vi "Display Biometry Ascan.vi"(8 "错误常量":errorcluster, 9 "L_Or_R":string, 10 "Measure_No":i32, 11 "connection reference":T1) -> (0 "error out":errorcluster)   [LabVIEW 2015, in "Browse.lvlib"]
uses:
  Browse.lvlib
  <vilib>/addons/database/Connection.llb/Conn ObjectReference.ctl
  Support/Display Biometry Ascan State.ctl
  Support/Biometry Ascan UI Data.ctl
  Sub VIs/Database Processing/Database Processing.lvlib
  Sub VIs/Utility VIs/Utility VIs.lvlib
  <vilib>/addons/database/NI_Database_API.lvlib
panel:
  out "Ascan":dbl[][](graph)
  out "Parameter":string[][](table)
  in  "停止按钮":bool
  out "状态栏":string
  # "眼轴参数"
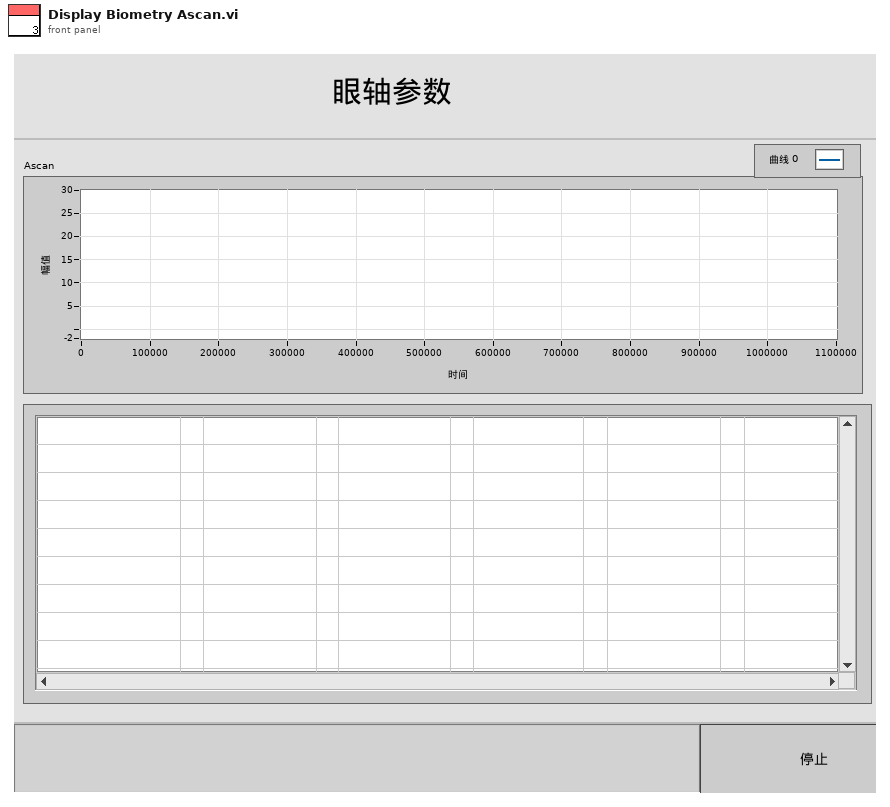
[diagram p1: front panel]
types:
  T1 = typedef "NI_Database_API.lvlib/Conn ObjectReference.ctl" = refnum<k1>
  T2 = typedef "Browse.lvlib/Biometry Ascan UI Data.ctl" = cluster{"Parameter引用句柄":refnum<vi>, "状态栏引用句柄":refnum<vi>, "退出引用句柄":refnum<vi>, "Asacn引用句柄":refnum<vi>}
  T3 = typedef "Browse.lvlib/Display Biometry Ascan State.ctl" = enum16{"Initialize", "Connect Database", "Update Biometry Ascan Single", "Update Biometry Ascan multiple", "Update Biometry Parameter", "Wait For Event", "Exit"}
  T4 = typedef "LVPoint32TypeDef.ctl" = cluster{"Horizontal":i32, "Vertical":i32}
  T5 = typedef "LVRowAndColumnTypeDef.ctl" = cluster{"Row":i32, "Column":i32}
  T6 = typedef "Database Processing.lvlib/Biometry Data Path.ctl" = cluster{"Measure_ID":i64, "Ascan_data_Original":string, "picture_pupil_Original":string, "picture_WTW_Original":string, "Ascan_data_Processing":string, "picture_pupil_Processing":string, "picture_WTW_Processing":string, "picture_Processing_K":string, "picture_Processing_ALL":string}
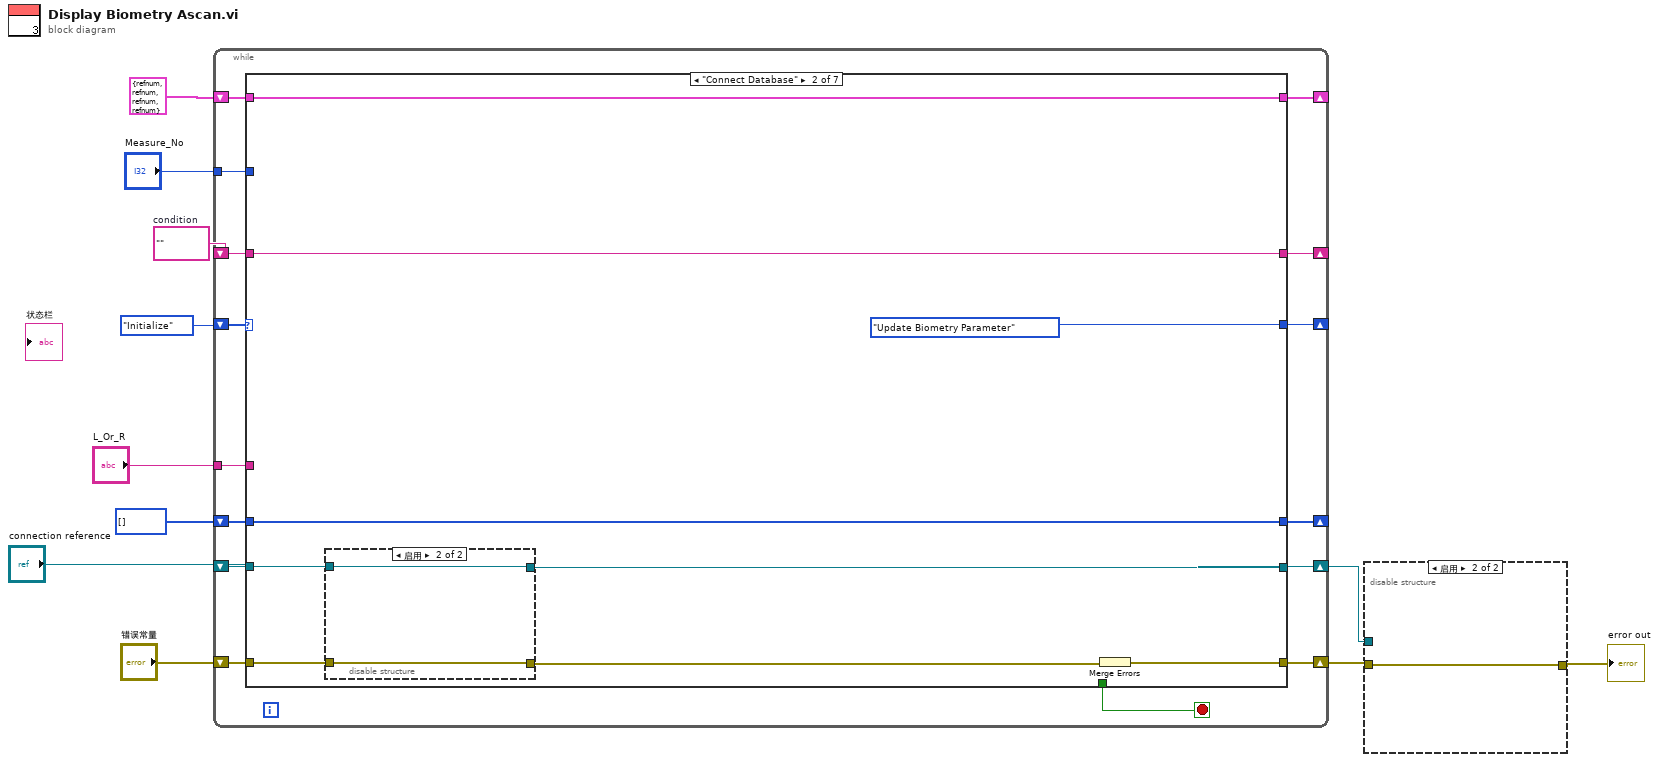
[diagram p0: block diagram]
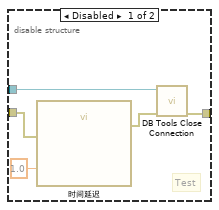
[diagram p2: hidden frame]
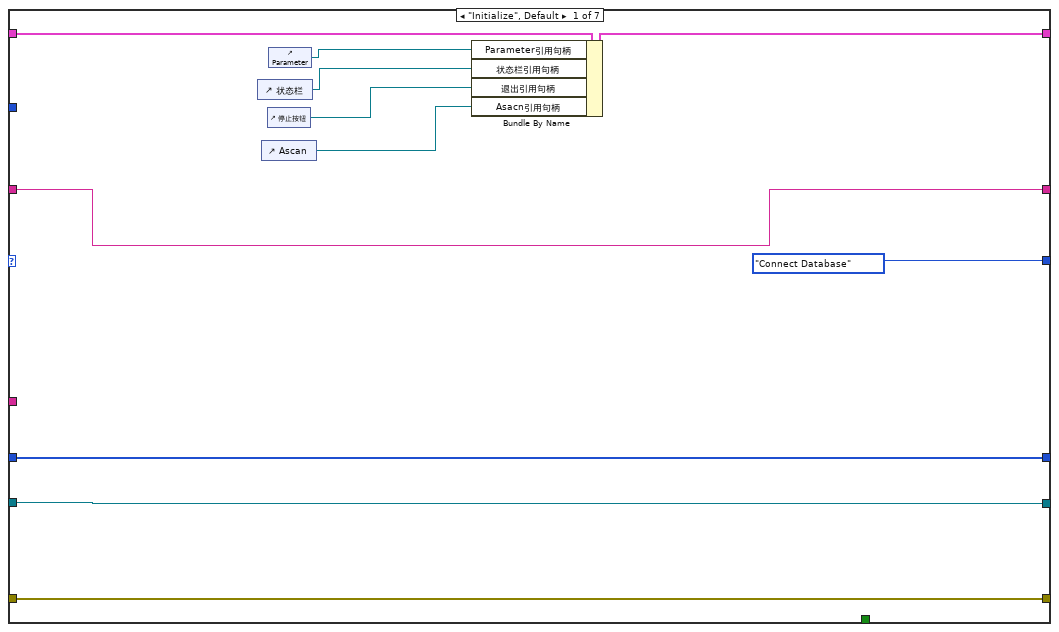
[diagram p3: hidden frame]
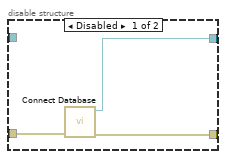
[diagram p4: hidden frame]
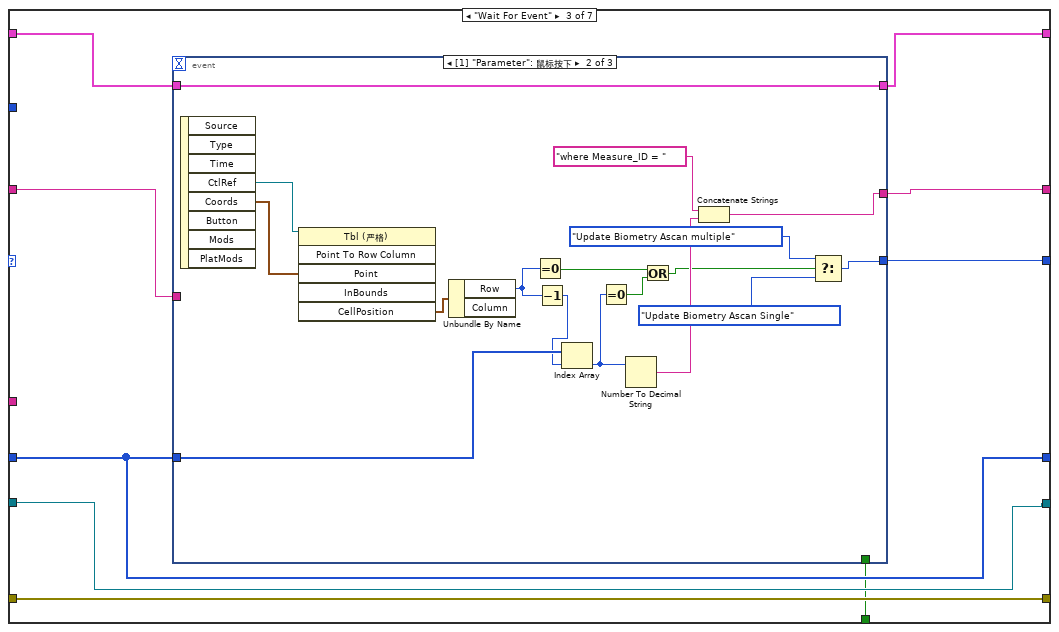
[diagram p5: hidden frame]
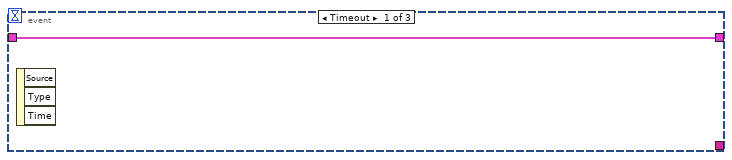
[diagram p6: hidden frame]
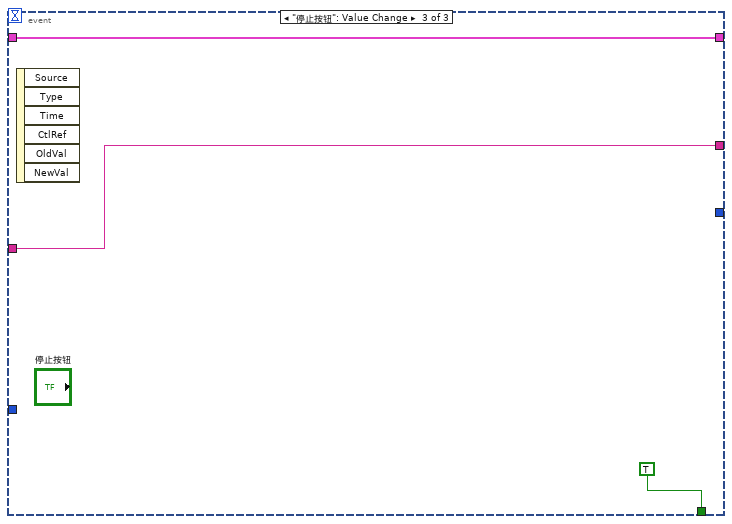
[diagram p7: hidden frame]
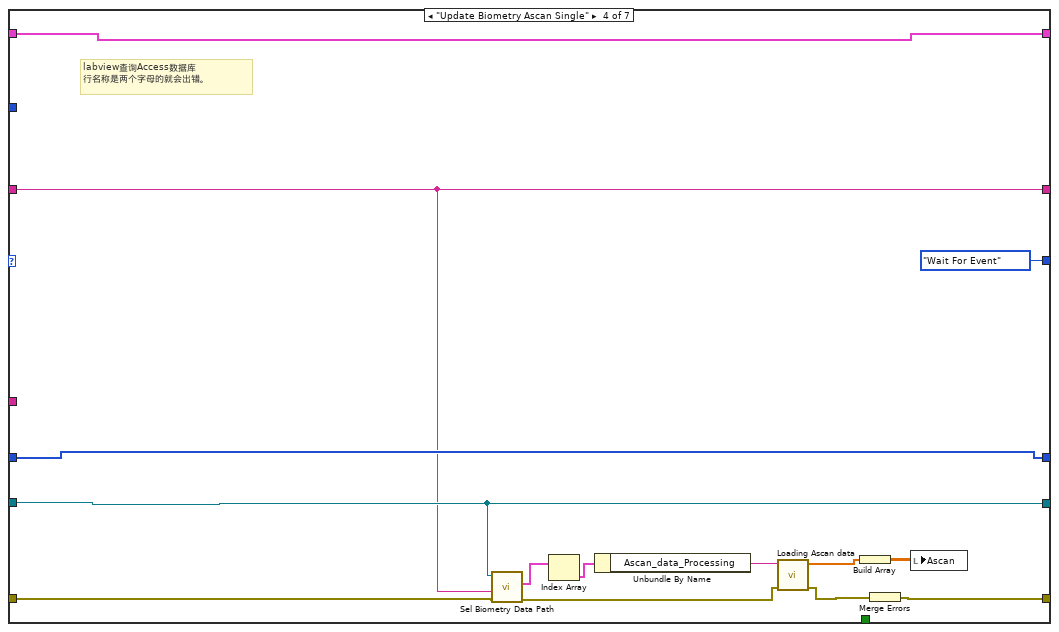
[diagram p8: hidden frame]
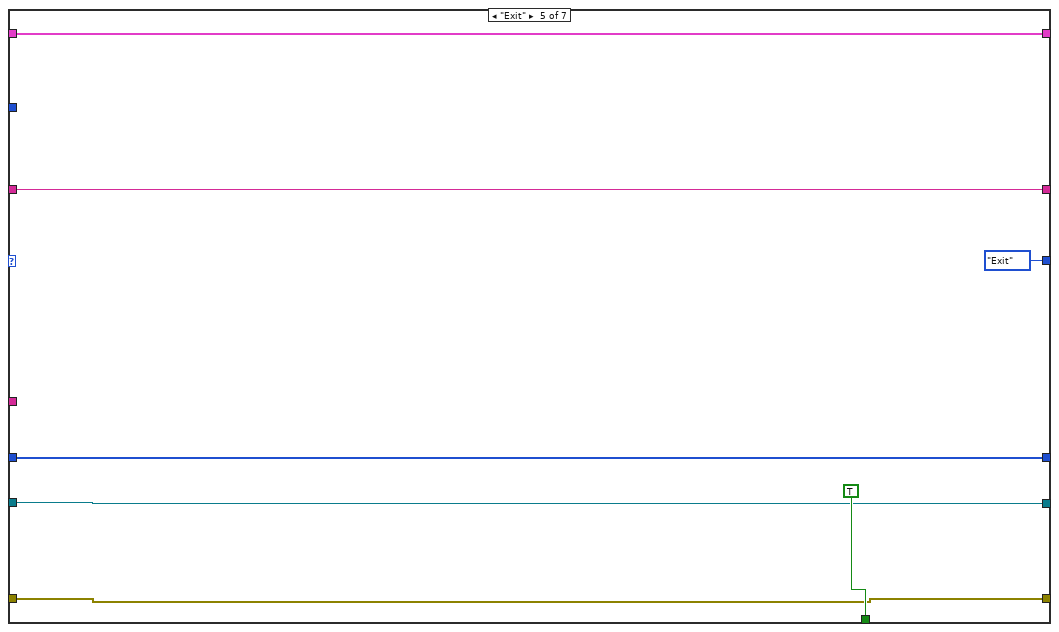
[diagram p9: hidden frame]
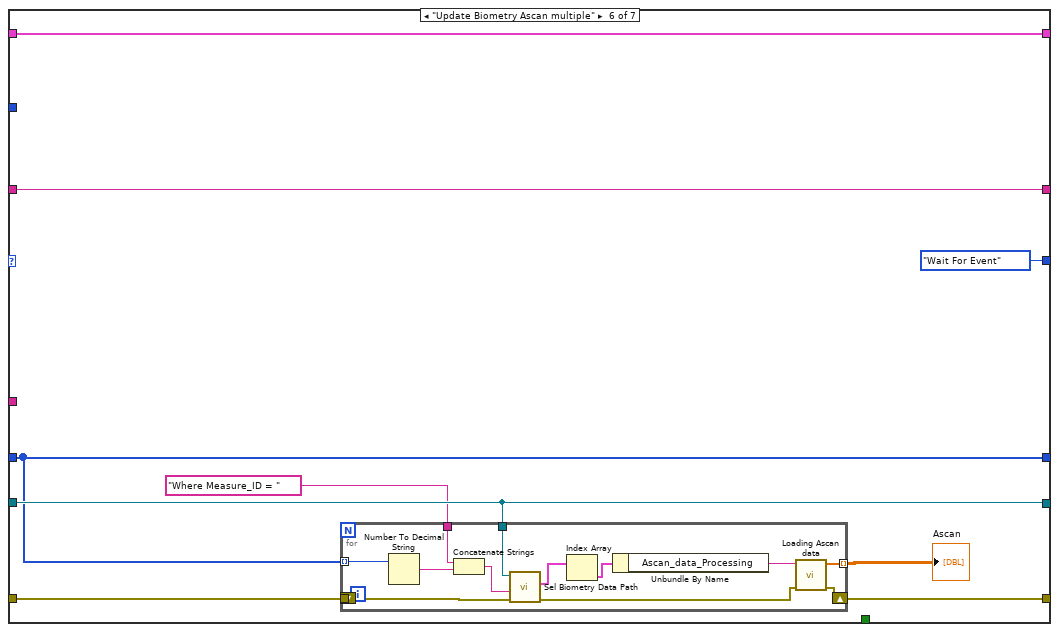
[diagram p10: hidden frame]
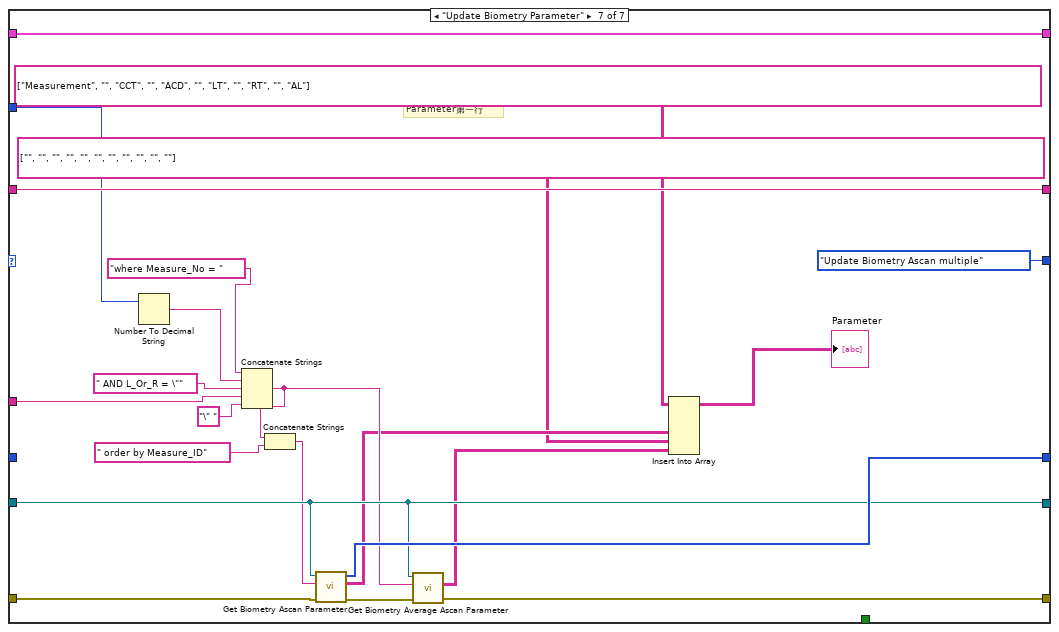
[diagram p11: hidden frame]
diagram:
  w9 = ""  # condition
  n1 = while {
    shift-right: [w25] -> _
    shift-left: T2 {"Parameter引用句柄"=refnum, "状态栏引用句柄"=refnum, "退出引用句柄"=refnum, "Asacn引用句柄"=refnum} ("UI数据") -> [w26]
    shift-right: [w17] -> _
    shift-left: Display_Biometry_Ascan_State."Initialize" ("State") -> [w16]
    shift-right: [w22] -> w3
    shift-left: "错误常量" -> [w24]
    shift-right: [w20] -> _
    shift-left: w9 -> [w23]
    shift-right: [w19] -> w1
    shift-left: "connection reference" -> [w18]
    shift-right: [w15] -> _
    shift-left: i64[] [] -> [w12]
    tunnel: "Measure_No" -> [w14]
    tunnel: "L_Or_R" -> [w13]
    stop <- w21 stop-if-true
    n2 = case shown="\"Connect Database\"" w16 {
      tunnel: w26 -> [w37 w41 w57 w94 w102 w111 w145]
      tunnel: [w36 w41 w56 w94 w102 w111 w145] -> w25
      tunnel: [Display_Biometry_Ascan_State."Connect Database" ("State") Display_Biometry_Ascan_State."Update Biometry Parameter" ("State") w55 Display_Biometry_Ascan_State."Wait For Event" ("State") Display_Biometry_Ascan_State."Exit" ("State") Display_Biometry_Ascan_State."Wait For Event" ("State") Display_Biometry_Ascan_State."Update Biometry Ascan multiple" ("State")] -> w17
      tunnel: w24 -> [w35 w45 w58 w86 w99 w106 w143]
      tunnel: w23 -> [w34 w42 w60 w84 w101 w110 w144]
      tunnel: [w35 w46 w58 w95 w99 w107 w127] -> w22
      tunnel: [w34 w42 w59 w84 w101 w110 w144] -> w20
      tunnel: [_ _ w52 _ TRUE _ _] -> w21
      tunnel: w18 -> [w33 w38 w53 w85 w98 w109 w135]
      tunnel: [w33 w43 w53 w85 w98 w109 w135] -> w19
      tunnel: [w31 w39 w54 w92 w97 w103 w142] -> w15
      tunnel: w14 -> [_ _ _ _ _ _ w141]
      tunnel: w13 -> [_ _ _ _ _ _ w139]
      tunnel: w12 -> [w31 w39 w54 w92 w97 w103 _]
      frame "Initialize", Default {
        n3 = control-ref of="状态栏"() -> (w29:refnum<vi>)
        n4 = control-ref of="Ascan"() -> (w27:refnum<vi>)
        n5 = control-ref of="停止按钮"() -> (w28:refnum<vi>)
        n6 = control-ref of="Parameter"() -> (w30:refnum<vi>)
        n7 = Bundle By Name(cluster=w37, "Parameter引用句柄"=w30, "状态栏引用句柄"=w29, "退出引用句柄"=w28, "Asacn引用句柄"=w27) -> (w36:T2)
      }
      frame "Connect Database" {
        n8 = disable-structure shown="启用" {
          disable-tunnel: w45 -> [w49 w50]
          disable-tunnel: [w48 w50] -> w44
          disable-tunnel: [w47 w51] -> w43
          disable-tunnel: w38 -> [_ w51]
          frame Disabled {
            n9 = call "Connect Database.vi"("error in (no error)"=w49) -> ("error out"=w48:errorcluster, "connection reference"=w47:T1)  [unwired: 9 in]
          }
          frame Enabled {
          }
        }
        n10 = Merge Errors(w44) -> (w46:errorcluster)
      }
      frame "Wait For Event" {
        n11 = event shown="[1] \"Parameter\": 鼠标按下" {
          selector: _ -> [_ _ _]
          dyn-events: _ -> [_ _ _]
          timeout: _ -> [_ _ _]
          tunnel: w60 -> [_ _ w81]
          tunnel: [_ w75 w81] -> w59
          tunnel: w57 -> [w61 w76 w80]
          tunnel: [w61 w76 w80] -> w56
          tunnel: w54 -> [_ w72 _]
          tunnel: [_ w62 _] -> w55
          tunnel: [_ _ TRUE] -> w52
          event Timeout {
            n12 = event-data() -> ()  [unwired: 1 in, 3 out]
          }
          event "Parameter": Mouse Down {
            n13 = event-data() -> ("CtlRef"=w73:refnum<vi>, "Coords"=w74:T4)  [unwired: 1 in, 6 out]
            n14 = invoke on="调用节点" class="Tbl (严格)" method="Point To Row Column"(reference=w73, "Point"=w74) -> ("CellPosition"=w78:T5)  [unwired: 4 in, 5 out]
            n15 = Unbundle By Name(w78) -> ("Row"=w68:i32)  [unwired: 1 out]
            n16 = Equal To 0?(x=w68) -> (x = 0?=w64:bool)
            n17 = Decrement(x=w68) -> (x-1=w67:i32)
            n18 = Index Array(array=w72, index=w67) -> (element=w66:i64)
            n19 = Equal To 0?(x=w66) -> (x = 0?=w65:bool)
            n20 = Number To Decimal String(number=w66) -> (decimal integer string=w71:string)  [unwired: 1 in]
            n21 = Or(x=w64, y=w65) -> (x .or. y?=w63:bool)
            n22 = Concatenate Strings("where Measure_ID = " ("字符串"), w71) -> (w75:string)
            n23 = Select(t=Display_Biometry_Ascan_State."Update Biometry Ascan multiple" ("State"), s=w63, f=Display_Biometry_Ascan_State."Update Biometry Ascan Single") -> (s? t:f=w62:T3)
          }
          event "停止按钮": Value Change {
            n24 = event-data() -> ()  [unwired: 1 in, 6 out]
          }
        }
      }
      frame "Update Biometry Ascan Single" {
        # "labview查询Access数据库\n行名称是两个字母的就会出错。"
        n25 = call "Sel Biometry Data Path.vi"("error in (no error)"=w86, "condition"=w84, "connection reference"=w85) -> ("error out"=w87:errorcluster, "Biometry Data Path"=w90:T6[])  [unwired: 7 in]
        n26 = Index Array(array=w90) -> (element=w89:T6)  [unwired: 1 in]
        n27 = Unbundle By Name(w89) -> ("Ascan_data_Processing"=w88:string)
        n28 = call "Loading Ascan data.vi"("error in (no error)"=w87, "名称或相对路径"=w88) -> ("error out"=w91:errorcluster, "first row"=w83:dbl[])  [unwired: 8 in]
        n29 = Build Array(w83) -> (w82:dbl[][])
        n30 = Merge Errors(w91) -> (w95:errorcluster)
        n31 = local write "Ascan"(w82) -> ()
      }
      frame "Exit" {
      }
      frame "Update Biometry Ascan multiple" {
        n32 = for {
          tunnel: w106 -> [w123]
          tunnel: w109 -> [w122]
          tunnel: w103 -> [w121] mode=indexing
          tunnel: "Where Measure_ID = " ("字符串") -> [w119]
          shift-right: [w113] -> w107
          shift-left: _ -> [_]
          tunnel: [w112] -> w105 mode=indexing
          n33 = Number To Decimal String(number=w121) -> (decimal integer string=w120:string)  [unwired: 1 in]
          n34 = Concatenate Strings(w119, w120) -> (w118:string)
          n35 = call "Sel Biometry Data Path.vi"("error in (no error)"=w123, "condition"=w118, "connection reference"=w122) -> ("error out"=w114:errorcluster, "Biometry Data Path"=w117:T6[])  [unwired: 7 in]
          n36 = Index Array(array=w117) -> (element=w116:T6)  [unwired: 1 in]
          n37 = Unbundle By Name(w116) -> ("Ascan_data_Processing"=w115:string)
          n38 = call "Loading Ascan data.vi"("error in (no error)"=w114, "名称或相对路径"=w115) -> ("error out"=w113:errorcluster, "first row"=w112:dbl[])  [unwired: 8 in]
        }
        "Ascan" <- w105
      }
      frame "Update Biometry Parameter" {
        # "Parameter第一行"
        n39 = Number To Decimal String(number=w141) -> (decimal integer string=w138:string)  [unwired: 1 in]
        n40 = Concatenate Strings("where Measure_No = " ("字符串"), w138, " AND L_Or_R = \"" ("字符串"), w139, "\" " ("字符串")) -> (w132:string)
        n41 = Concatenate Strings(w132, " order by Measure_ID" ("字符串")) -> (w133:string)
        n42 = call "Get Biometry Ascan Parameter.vi"("error in (no error)"=w143, "condition"=w133, "connection reference"=w135) -> ("error out"=w136:errorcluster, "Data Output"=w130:string[][], "Measure_ID"=w142:i64[])  [unwired: 6 in]
        n43 = call "Get Biometry Average Ascan Parameter.vi"("error in (no error)"=w136, "condition"=w132, "connection reference"=w135) -> ("error out"=w127:errorcluster, "Data Output"=w125:string[][])  [unwired: 7 in]
        n44 = Insert Into Array(array=string[][] [["Measurement", "", "CCT", "", "ACD", "", "LT", "", "RT", "", "AL"]], new element #1=w130, new element #2=string[][] [["", "", "", "", "", "", "", "", "", "", ""]], new element #3=w125) -> (→"Parameter":string[][])  [unwired: 2 in]
      }
    }
  }
  n45 = disable-structure shown="启用" {
    disable-tunnel: w3 -> [w148 w151]
    disable-tunnel: [w150 w151] -> w2
    disable-tunnel: w1 -> [w149 _]
    frame Disabled {
      # "Test"
      n46 = call "时间延迟"("error in (no error)"=w148, "Delay Time (s)"=1.0) -> ("error out"=w147:errorcluster)  [unwired: 9 in]
      n47 = call <vilib>:"DB Tools Close Connection.vi"("error in (no error)"=w147, "connection reference"=w149) -> ("error out"=w150:errorcluster)  [unwired: 5 in]
    }
    frame Enabled {
    }
  }
  "error out" <- w2
